vi "Set Duty Cycle and Frequency.vi"(7 "error in (no error)":errorcluster, 8 "Frequency [Hz]":dbl=1000.0, 9 "Duty Cycle":dbl=0.5, 10 "PWM Ref In":T1) -> (0 "error out":errorcluster, 3 "PWM Ref Out":T1)   [LabVIEW 2021, in "PWM.lvlib"]
doc: "Sets the duty cycle value and frequency value of a pulse width modulation (PWM) signal."
uses:
  <vilib>/myRIO/Instrument Drivers/Onboard IO/PWM/PWM.lvlib
  <vilib>/myRIO/Instrument Drivers/Onboard IO/PWM/typedefs/PWM Reference.ctl
  <vilib>/myRIO/Common/Instrument Driver Framework/Utilities/typedefs/myRIO Generic Hardware Reference.ctl
  <vilib>/myRIO/Common/Instrument Driver Framework/Utilities/typedefs/Hardware Version Enum.ctl
  <vilib>/myRIO/Common/Instrument Driver Framework/Utilities/typedefs/myRIO v1.0 Reference.ctl
  <vilib>/myRIO/Common/Instrument Driver Framework/Utilities/typedefs/Generic FPGA Reference.ctl
  <vilib>/myRIO/Common/Instrument Driver Framework/myRIO v1.0/PWM/typedefs/PWM Channels Enum.ctl
  <vilib>/myRIO/Instrument Drivers/Onboard IO/PWM/typedefs/PWM Configuration.ctl
  <vilib>/myRIO/Common/Instrument Driver Framework/myRIO v1.0/PWM/typedefs/PWM Configuration v1.0.ctl
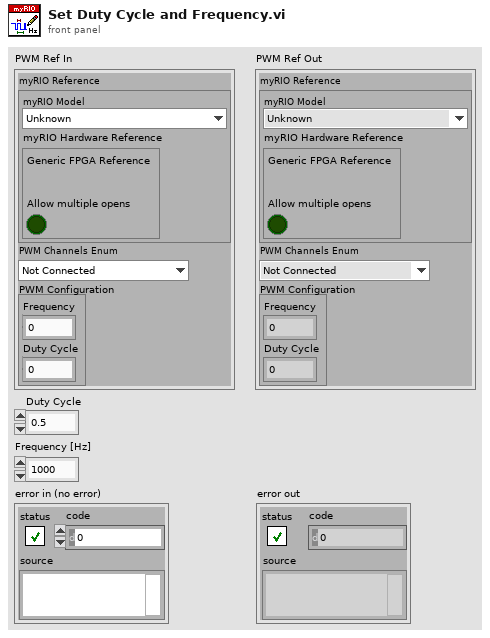
[diagram p1: front panel]
types:
  T1 = typedef "PWM.lvlib/PWM Reference.ctl" = cluster{"myRIO Reference":T2, "PWM Channels Enum":T6, "PWM Configuration":T7}
  T2 = typedef "myRIO Generic Hardware Reference.ctl" = cluster{"myRIO Model":T3, "myRIO Hardware Reference":T4}
  T3 = typedef "Hardware Version Enum.ctl" = enum16{"Unknown", "myRIO-1900", "myRIO-1950", "roboRIO", "NI ELVIS RIO CM", "ELVIS III"}
  T4 = typedef "myRIO v1.0 Reference.ctl" = cluster{"Generic FPGA Reference":T5, "Allow multiple opens":bool}
  T5 = typedef "Generic FPGA Reference.ctl" = refnum<k20>
  T6 = typedef "PWM Channels Enum.ctl" = enum16{"Not Connected", "C/PWM0", "C/PWM1", "A/PWM0", "A/PWM1", "A/PWM2", "A/PWM3", "A/PWM4", "A/PWM5", "A/PWM6", "A/PWM7", "A/PWM8", "A/PWM9", "A/PWM10", "A/PWM11", "A/PWM12", "A/PWM13", "A/PWM14", "A/PWM15", "A/PWM16", "A/PWM17", "A/PWM18", "A/PWM19", "B/PWM0", "B/PWM1", "B/PWM2", "B/PWM3", "B/PWM4", "B/PWM5", "B/PWM6", "B/PWM7", "B/PWM8", "B/PWM9", "B/PWM10", "B/PWM11", "B/PWM12", "B/PWM13", "B/PWM14", "B/PWM15", "B/PWM16", "B/PWM17", "B/PWM18", "B/PWM19", "PWM/PWM0", "PWM/PWM1", "PWM/PWM2", "PWM/PWM3", "PWM/PWM4", "PWM/PWM5", "PWM/PWM6", "PWM/PWM7", "PWM/PWM8", "PWM/PWM9"}
  T7 = typedef "PWM.lvlib/PWM Configuration.ctl" = cluster{"Frequency":dbl, "Duty Cycle":dbl}
  T8 = typedef "PWM Configuration v1.0.ctl" = cluster{"Frequency (Hz)":dbl, "Duty Cycle":dbl}
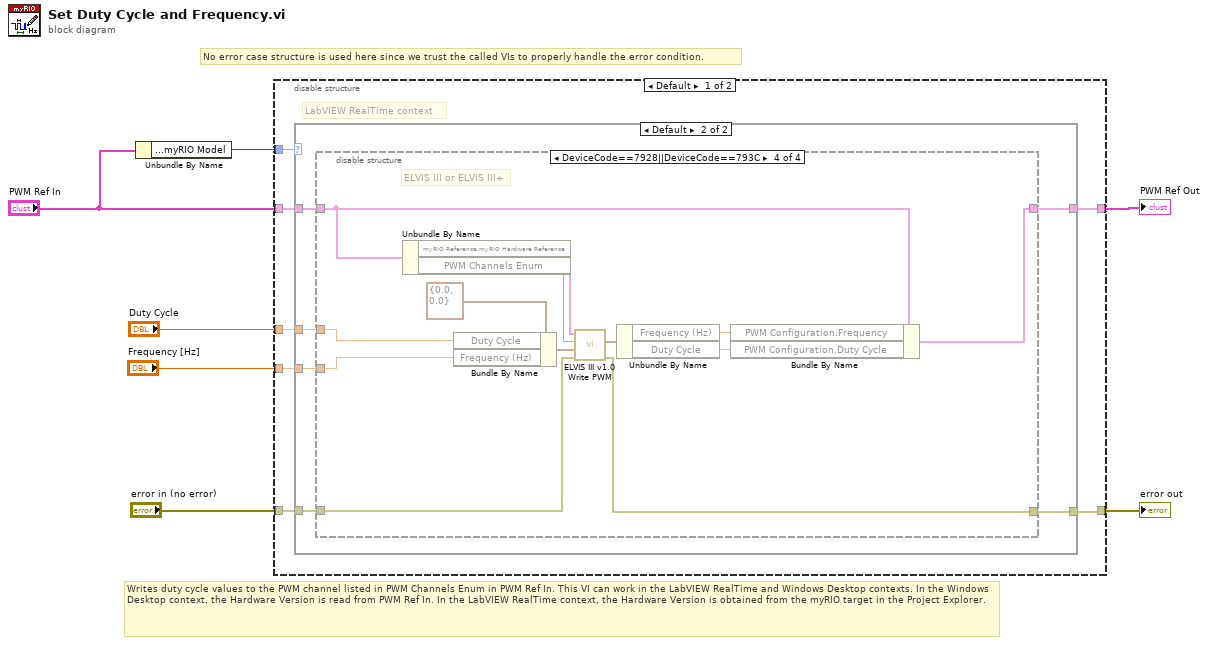
[diagram p0: block diagram]
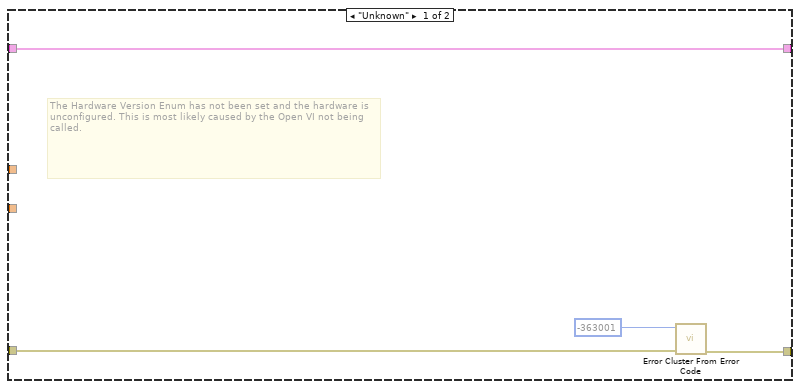
[diagram p2: hidden frame]
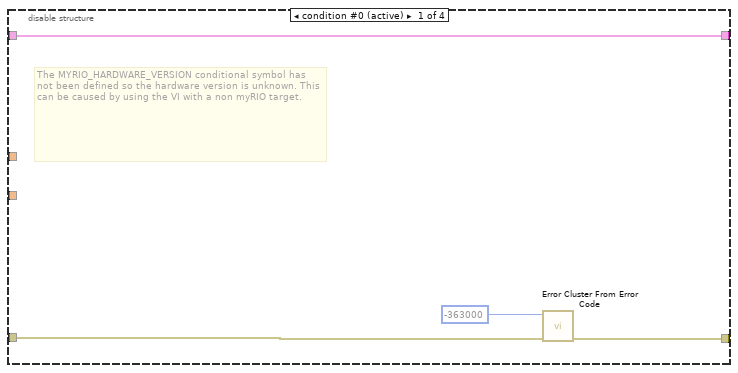
[diagram p3: hidden frame]
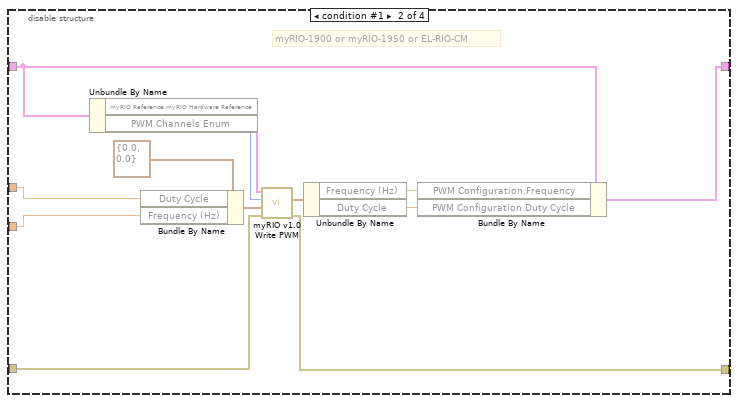
[diagram p4: hidden frame]
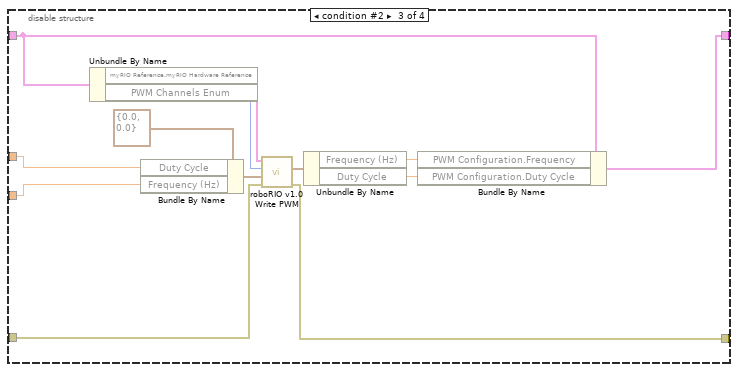
[diagram p5: hidden frame]
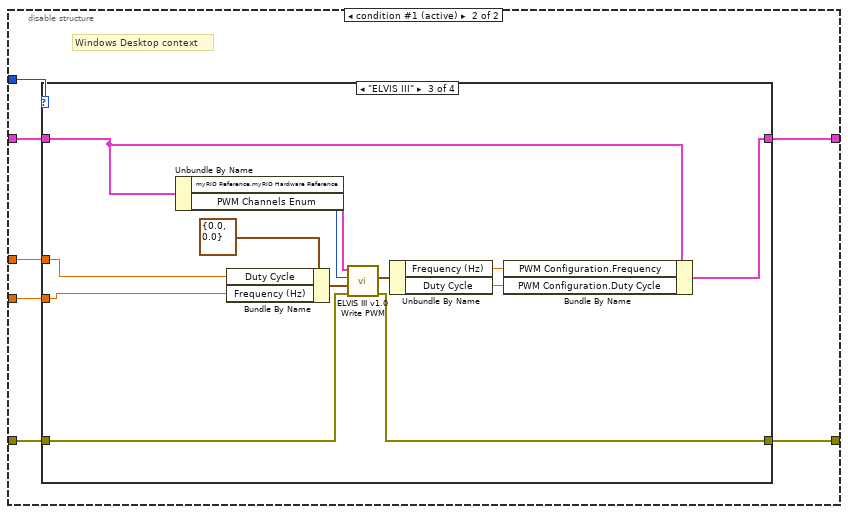
[diagram p6: hidden frame]
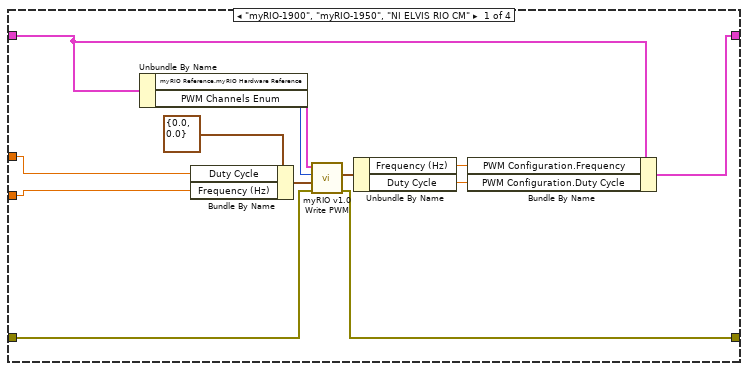
[diagram p7: hidden frame]
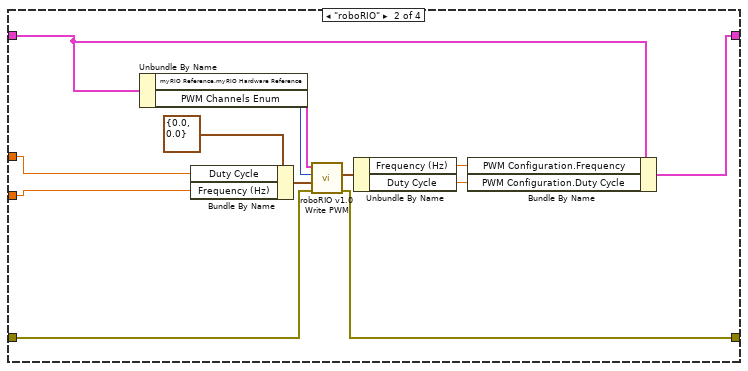
[diagram p8: hidden frame]
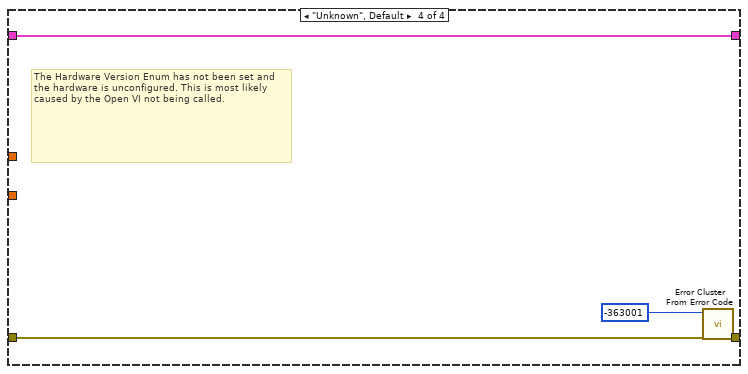
[diagram p9: hidden frame]
diagram:
  # "No error case structure is used here since we trust the called VIs to properly handle the error condition."
  # "Writes duty cycle values to the PWM channel listed in PWM Channels Enum in PWM Ref In. This VI can work in the LabVIEW RealTime and Windows Desktop contexts. In the Windows Desktop context, the Hardware Version is read from PWM Ref In. In the LabVIEW RealTime context, the Hardware Version is obtained from the myRIO target in the Project Explorer."
  n1 = Unbundle By Name("PWM Ref In") -> ("myRIO Reference.myRIO Model"=w3:T3)
  n2 = disable-structure shown="Default" {
    disable-tunnel: [w14 w74] -> w4
    disable-tunnel: "PWM Ref In" -> [w13 w71]
    disable-tunnel: "error in (no error)" -> [w12 w73]
    disable-tunnel: [w11 w72] -> w5
    disable-tunnel: w3 -> [w10 w70]
    disable-tunnel: "Frequency [Hz]" -> [w8 w69]
    disable-tunnel: "Duty Cycle" -> [w9 w68]
    frame condition #0 {
      # "LabVIEW RealTime context"
      n3 = case shown="Default" w10 {
        tunnel: [w17 w24] -> w14
        tunnel: w13 -> [w15 w23]
        tunnel: w12 -> [w16 w22]
        tunnel: [w15 w21] -> w11
        tunnel: w9 -> [_ w20]
        tunnel: w8 -> [_ w19]
        frame "Unknown" {
          # "The Hardware Version Enum has not been set and the hardware is unconfigured. This is most likely caused by the Open VI not being called."
          n4 = call <vilib>:"Error Cluster From Error Code.vi"("error in (no error)"=w16, "error code (0)"=-363001) -> ("error out"=w17:errorcluster)  [unwired: 7 in]
        }
        frame Default {
          n5 = disable-structure shown="DeviceCode==7928||DeviceCode==793C" {
            disable-tunnel: w23 -> [w25 w33 w46 w59]
            disable-tunnel: [w28 w29 w42 w55] -> w24
            disable-tunnel: w22 -> [w26 w32 w45 w56]
            disable-tunnel: [w25 w34 w47 w60] -> w21
            disable-tunnel: w20 -> [_ w31 w44 w58]
            disable-tunnel: w19 -> [_ w30 w43 w57]
            frame condition #0 (active) {
              # "The MYRIO_HARDWARE_VERSION conditional symbol has not been defined so the hardware version is unknown. This can be caused by using the VI with a non myRIO target."
              n6 = call <vilib>:"Error Cluster From Error Code.vi"("error in (no error)"=w26, "error code (0)"=-363000) -> ("error out"=w28:errorcluster)  [unwired: 7 in]
            }
            frame condition #1 {
              # "myRIO-1900 or myRIO-1950 or EL-RIO-CM"
              n7 = Unbundle By Name(w33) -> ("myRIO Reference.myRIO Hardware Reference"=w41:T4, "PWM Channels Enum"=w40:T6)
              n8 = Bundle By Name(cluster=T8 {"Frequency (Hz)"=0.0, "Duty Cycle"=0.0} ("PWM Configuration"), "Duty Cycle"=w31, "Frequency (Hz)"=w30) -> (w38:T8)
              n9 = call <vilib>:"myRIO v1.0 Write PWM.vi"("error in (no error)"=w32, "PWM Configuration In"=w38, "Channel"=w40, "myRIO Ref In"=w41) -> ("error out"=w29:errorcluster, "PWM Configuration Out"=w37:T8)  [unwired: 5 in, 1 out]
              n10 = Unbundle By Name(w37) -> ("Frequency (Hz)"=w36:dbl, "Duty Cycle"=w35:dbl)
              n11 = Bundle By Name(cluster=w33, "PWM Configuration.Frequency"=w36, "PWM Configuration.Duty Cycle"=w35) -> (w34:T1)
            }
            frame condition #2 {
              n12 = Unbundle By Name(w46) -> ("myRIO Reference.myRIO Hardware Reference"=w54:T4, "PWM Channels Enum"=w53:T6)
              n13 = Bundle By Name(cluster=T8 {"Frequency (Hz)"=0.0, "Duty Cycle"=0.0} ("PWM Configuration"), "Duty Cycle"=w44, "Frequency (Hz)"=w43) -> (w51:T8)
              n14 = call <vilib>:"roboRIO v1.0 Write PWM.vi"("error in (no error)"=w45, "PWM Configuration In"=w51, "Channel"=w53, "myRIO Ref In"=w54) -> ("error out"=w42:errorcluster, "PWM Configuration Out"=w50:T8)  [unwired: 5 in, 1 out]
              n15 = Unbundle By Name(w50) -> ("Frequency (Hz)"=w49:dbl, "Duty Cycle"=w48:dbl)
              n16 = Bundle By Name(cluster=w46, "PWM Configuration.Frequency"=w49, "PWM Configuration.Duty Cycle"=w48) -> (w47:T1)
            }
            frame condition #3 {
              # "ELVIS III or ELVIS III+"
              n17 = Unbundle By Name(w59) -> ("myRIO Reference.myRIO Hardware Reference"=w67:T4, "PWM Channels Enum"=w66:T6)
              n18 = Bundle By Name(cluster=T8 {"Frequency (Hz)"=0.0, "Duty Cycle"=0.0} ("PWM Configuration"), "Duty Cycle"=w58, "Frequency (Hz)"=w57) -> (w64:T8)
              n19 = call <vilib>:"ELVIS III v1.0 Write PWM.vi"("error in (no error)"=w56, "PWM Configuration In"=w64, "Channel"=w66, "myRIO Ref In"=w67) -> ("error out"=w55:errorcluster, "PWM Configuration Out"=w63:T8)  [unwired: 5 in, 1 out]
              n20 = Unbundle By Name(w63) -> ("Frequency (Hz)"=w62:dbl, "Duty Cycle"=w61:dbl)
              n21 = Bundle By Name(cluster=w59, "PWM Configuration.Frequency"=w62, "PWM Configuration.Duty Cycle"=w61) -> (w60:T1)
            }
          }
        }
      }
    }
    frame condition #1 (active) {
      # "Windows Desktop context"
      n22 = case shown="\"ELVIS III\"" w70 {
        tunnel: [w75 w88 w102 w117] -> w74
        tunnel: w71 -> [w80 w93 w106 w114]
        tunnel: w73 -> [w77 w90 w103 w115]
        tunnel: [w76 w89 w101 w114] -> w72
        tunnel: w69 -> [w78 w91 w104 _]
        tunnel: w68 -> [w79 w92 w105 _]
        frame "myRIO-1900", "myRIO-1950", "NI ELVIS RIO CM" {
          n23 = Unbundle By Name(w80) -> ("myRIO Reference.myRIO Hardware Reference"=w87:T4, "PWM Channels Enum"=w86:T6)
          n24 = Bundle By Name(cluster=T8 {"Frequency (Hz)"=0.0, "Duty Cycle"=0.0} ("PWM Configuration"), "Duty Cycle"=w79, "Frequency (Hz)"=w78) -> (w84:T8)
          n25 = call <vilib>:"myRIO v1.0 Write PWM.vi"("error in (no error)"=w77, "PWM Configuration In"=w84, "Channel"=w86, "myRIO Ref In"=w87) -> ("error out"=w75:errorcluster, "PWM Configuration Out"=w83:T8)  [unwired: 5 in, 1 out]
          n26 = Unbundle By Name(w83) -> ("Frequency (Hz)"=w82:dbl, "Duty Cycle"=w81:dbl)
          n27 = Bundle By Name(cluster=w80, "PWM Configuration.Frequency"=w82, "PWM Configuration.Duty Cycle"=w81) -> (w76:T1)
        }
        frame "roboRIO" {
          n28 = Unbundle By Name(w93) -> ("myRIO Reference.myRIO Hardware Reference"=w100:T4, "PWM Channels Enum"=w99:T6)
          n29 = Bundle By Name(cluster=T8 {"Frequency (Hz)"=0.0, "Duty Cycle"=0.0} ("PWM Configuration"), "Duty Cycle"=w92, "Frequency (Hz)"=w91) -> (w97:T8)
          n30 = call <vilib>:"roboRIO v1.0 Write PWM.vi"("error in (no error)"=w90, "PWM Configuration In"=w97, "Channel"=w99, "myRIO Ref In"=w100) -> ("error out"=w88:errorcluster, "PWM Configuration Out"=w96:T8)  [unwired: 5 in, 1 out]
          n31 = Unbundle By Name(w96) -> ("Frequency (Hz)"=w95:dbl, "Duty Cycle"=w94:dbl)
          n32 = Bundle By Name(cluster=w93, "PWM Configuration.Frequency"=w95, "PWM Configuration.Duty Cycle"=w94) -> (w89:T1)
        }
        frame "ELVIS III" {
          n33 = Unbundle By Name(w106) -> ("myRIO Reference.myRIO Hardware Reference"=w113:T4, "PWM Channels Enum"=w112:T6)
          n34 = Bundle By Name(cluster=T8 {"Frequency (Hz)"=0.0, "Duty Cycle"=0.0} ("PWM Configuration"), "Duty Cycle"=w105, "Frequency (Hz)"=w104) -> (w110:T8)
          n35 = call <vilib>:"ELVIS III v1.0 Write PWM.vi"("error in (no error)"=w103, "PWM Configuration In"=w110, "Channel"=w112, "myRIO Ref In"=w113) -> ("error out"=w102:errorcluster, "PWM Configuration Out"=w109:T8)  [unwired: 5 in, 1 out]
          n36 = Unbundle By Name(w109) -> ("Frequency (Hz)"=w108:dbl, "Duty Cycle"=w107:dbl)
          n37 = Bundle By Name(cluster=w106, "PWM Configuration.Frequency"=w108, "PWM Configuration.Duty Cycle"=w107) -> (w101:T1)
        }
        frame "Unknown", Default {
          # "The Hardware Version Enum has not been set and the hardware is unconfigured. This is most likely caused by the Open VI not being called."
          n38 = call <vilib>:"Error Cluster From Error Code.vi"("error in (no error)"=w115, "error code (0)"=-363001) -> ("error out"=w117:errorcluster)  [unwired: 7 in]
        }
      }
    }
  }
  "PWM Ref Out" <- w5
  "error out" <- w4
